vi "Get name.vi"(8 "Error in":errorcluster, 10 "Vi Path":path, 11 "LV MDI in":refnum<class "LV MDI.lvclass">) -> (0 "Error Out":errorcluster, 3 "LV MDI out":refnum<class "LV MDI.lvclass">)   [LabVIEW 2016, in "LV MDI.lvclass"]
uses:
  LV MDI.lvclass
  LV MDI.lvclass/LV MDI.ctl
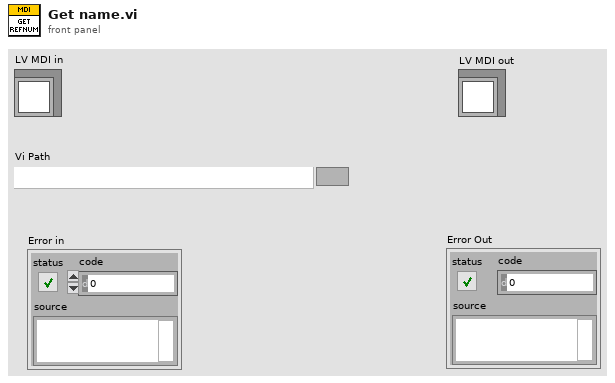
[diagram p1: front panel]
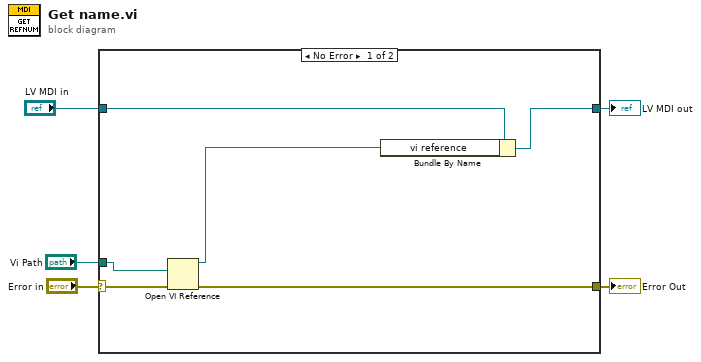
[diagram p0: block diagram]
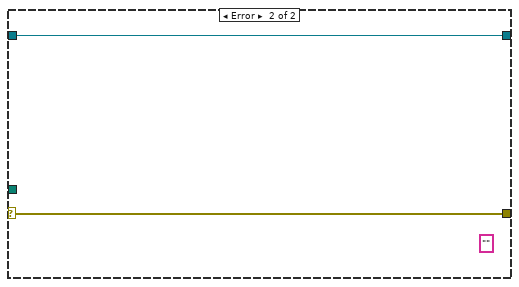
[diagram p2: hidden frame]
diagram:
  n1 = case shown="No Error" "Error in" {
    selector: "Error in" -> [w11 w13]
    tunnel: [w10 w13] -> w4
    tunnel: "Vi Path" -> [w9 _]
    tunnel: "LV MDI in" -> [w8 w12]
    tunnel: [w7 w12] -> w1
    frame No Error {
      n2 = Open VI Reference(vi path=w9, error in (no error)=w11) -> (vi reference=w6:refnum<vi>, error out=w10:errorcluster)  [unwired: 4 in]
      n3 = Bundle By Name(cluster=w8, "vi reference"=w6) -> (w7:refnum<class "LV MDI.lvclass">)
    }
    frame Error {
      (unwired) "" ("Front Panel.Title")
    }
  }
  "Error Out" <- w4
  "LV MDI out" <- w1
